vi "zad_13.vi"() -> ()   [LabVIEW 2024]
uses:
  State_13.ctl
  DataInfo_13.ctl
panel:
  out "Info":T1
  out "error out":errorcluster
  in  "error in":errorcluster
  in  "Stop":bool
  in  "Run cleaning":bool
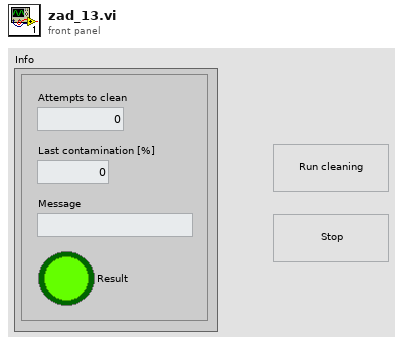
[diagram p1: front panel]
types:
  T1 = cluster{"Attempts to clean":dbl, "Last contamination [%]":dbl, "Message":string, "Result":bool}
  T2 = typedef "State_13.ctl" = enum16{"Init", "Idle", "Check", "Clean", "Stop", "Error"}
  T3 = typedef "DataInfo_13.ctl" = cluster{"Attempts to clean":dbl, "Last contamination [%]":dbl, "Message":string, "Result":bool}
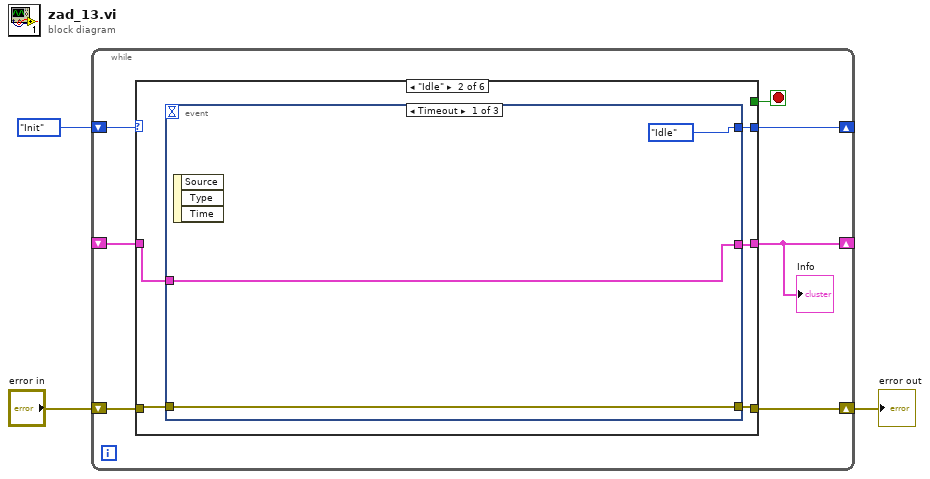
[diagram p0: block diagram]
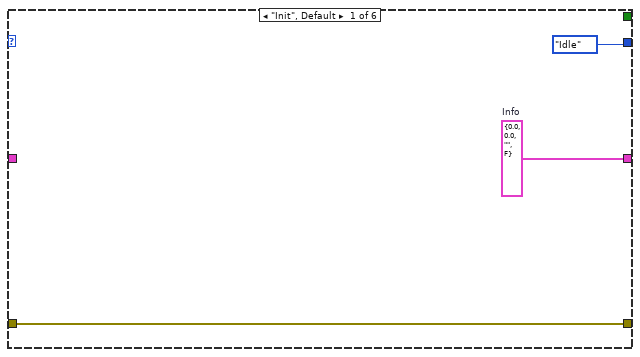
[diagram p2: hidden frame]
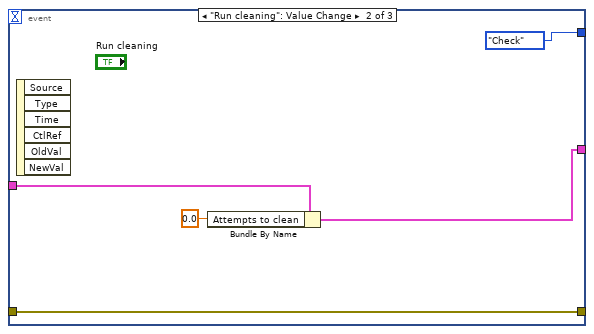
[diagram p3: hidden frame]
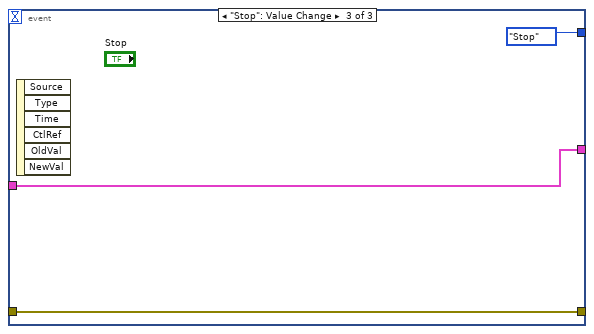
[diagram p4: hidden frame]
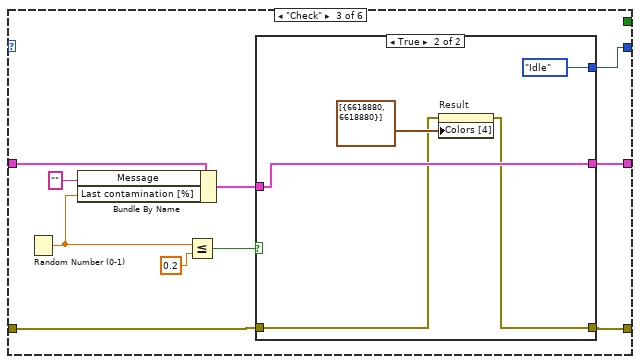
[diagram p5: hidden frame]
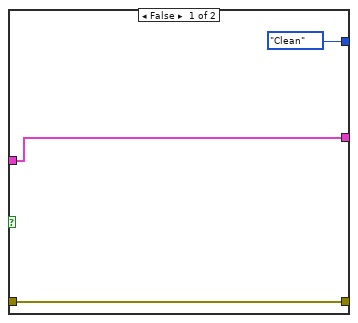
[diagram p6: hidden frame]
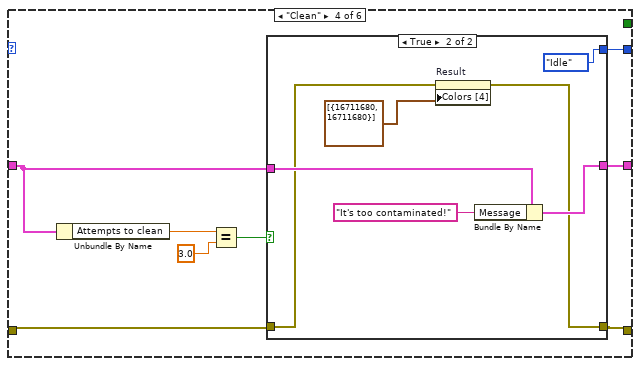
[diagram p7: hidden frame]
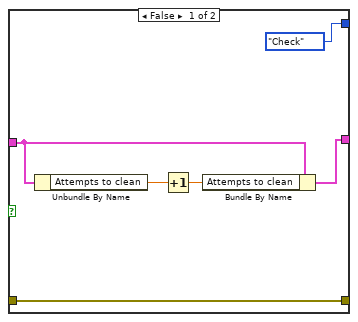
[diagram p8: hidden frame]
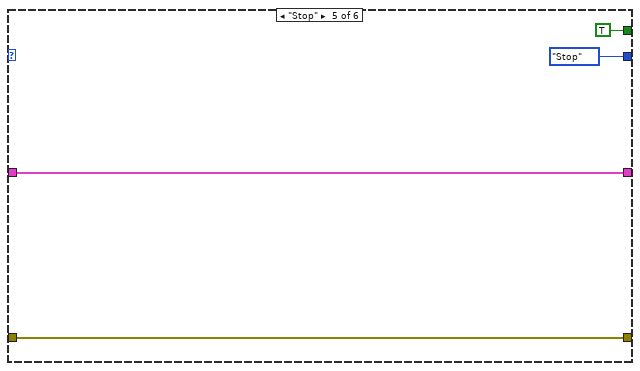
[diagram p9: hidden frame]
diagram:
  n1 = while {
    shift-right: [w8] -> _
    shift-left: State_13."Init" -> [w10]
    shift-right: [w7] -> w2
    shift-left: "error in" -> [w6]
    shift-right: [w4] -> _
    shift-left: _ -> [w5]
    stop <- w9 stop-if-true
    n2 = case shown="\"Idle\"" w10 {
      selector: w10 -> [_ _ _ _ _ w73]
      tunnel: [_ _ _ _ TRUE _] -> w9
      tunnel: [State_13."Idle" w14 w30 w53 State_13."Stop" w73] -> w8
      tunnel: [w13 w16 w39 w55 w70 w75] -> w7
      tunnel: w6 -> [w13 w15 w38 w54 w70 w75]
      tunnel: [w11 w18 w31 w48 w69 w74] -> w4
      tunnel: w5 -> [_ w17 w37 w49 w69 w74]
      frame "Init", Default {
        w11 = T3 {"Attempts to clean"=0.0, "Last contamination [%]"=0.0, "Message"="", "Result"=FALSE}  # Info
      }
      frame "Idle" {
        n3 = event shown="[0] Timeout" {
          selector: _ -> [_ _ _]
          dyn-events: _ -> [_ _ _]
          timeout: _ -> [_ _ _]
          tunnel: [w21 w23 w29] -> w18
          tunnel: w17 -> [w21 w24 w29]
          tunnel: [w20 w26 w28] -> w16
          tunnel: w15 -> [w20 w26 w28]
          tunnel: [State_13."Idle" State_13."Check" State_13."Stop"] -> w14
          event Timeout {
            n4 = event-data() -> ()  [unwired: 1 in, 3 out]
          }
          event "Run cleaning": Value Change {
            n5 = event-data() -> ()  [unwired: 1 in, 6 out]
            n6 = Bundle By Name(cluster=w24, "Attempts to clean"=0.0) -> (w23:T3)
          }
          event "Stop": Value Change {
            n7 = event-data() -> ()  [unwired: 1 in, 6 out]
          }
        }
      }
      frame "Check" {
        n8 = Random Number (0-1)() -> (number: 0 to 1=w35:dbl)
        n9 = Bundle By Name(cluster=w37, "Message"="", "Last contamination [%]"=w35) -> (w32:T3)
        n10 = Less Or Equal?(x=w35, y=0.2) -> (x <= y?=w33:bool)
        n11 = case shown="True" w33 {
          tunnel: [w42 w43] -> w39
          tunnel: w38 -> [w42 w44]
          tunnel: w32 -> [w41 w45]
          tunnel: [w41 w45] -> w31
          tunnel: [State_13."Clean" State_13."Idle"] -> w30
          frame False {
          }
          frame True {
            n12 = property on="Result" class="Boolean (strict)"(error in=w44, "Colors [4]"=cluster{u32, u32}[] [{6618880, 6618880}]) -> (error out=w43:errorcluster)  [unwired: 1 in, 1 out]
          }
        }
      }
      frame "Clean" {
        n13 = Unbundle By Name(w49) -> ("Attempts to clean"=w52:dbl)
        n14 = Equal?(x=w52, y=3.0) -> (x = y?=w50:bool)
        n15 = case shown="True" w50 {
          tunnel: [w61 w63] -> w55
          tunnel: w54 -> [w61 w62]
          tunnel: [State_13."Check" State_13."Idle"] -> w53
          tunnel: w49 -> [w59 w66]
          tunnel: [w58 w64] -> w48
          frame False {
            n16 = Unbundle By Name(w59) -> ("Attempts to clean"=w57:dbl)
            n17 = Increment(x=w57) -> (x+1=w56:dbl)
            n18 = Bundle By Name(cluster=w59, "Attempts to clean"=w56) -> (w58:T3)
          }
          frame True {
            n19 = property on="Result" class="Boolean (strict)"(error in=w62, "Colors [4]"=cluster{u32, u32}[] [{16711680, 16711680}]) -> (error out=w63:errorcluster)  [unwired: 1 in, 1 out]
            n20 = Bundle By Name(cluster=w66, "Message"="It's too contaminated!") -> (w64:T3)
          }
        }
      }
      frame "Stop" {
      }
      frame "Error" {
      }
    }
    "Info" <- w4
  }
  "error out" <- w2
